vi "isValidCH.vi"(8 "error in":errorcluster, 10 "ValidCh":T2[](array[typedef]) items=["7"=7, "11"=11, "12"=12, "13"=13, "15"=15, "16"=16, "18"=18, "29"=29, "32"=32, "33"=33, "35"=35, "36"=36, "37"=37, "38"=38, "40"=40], 11 "CHStIn":T1) -> (0 "error out":errorcluster, 3 "VaildCH?":bool)   [LabVIEW 2014, in "ValveCTRL.lvlib"]
uses:
  ValveCTRL.lvlib
  TypeDef/CHs_List.ctl
  TypeDef/ChannelStatus.ctl
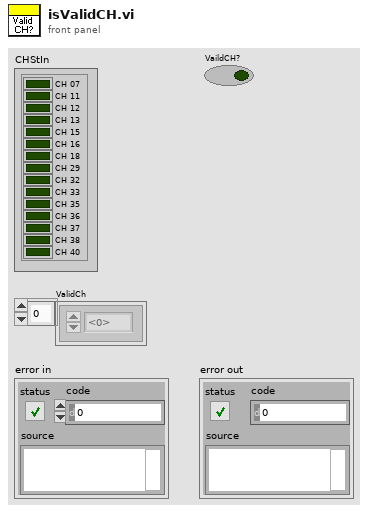
[diagram p1: front panel]
types:
  T1 = typedef "ValveCTRL.lvlib/ChannelStatus.ctl" = cluster{"CH 07":bool, "CH 11":bool, "CH 12":bool, "CH 13":bool, "CH 15":bool, "CH 16":bool, "CH 18":bool, "CH 29":bool, "CH 32":bool, "CH 33":bool, "CH 35":bool, "CH 36":bool, "CH 37":bool, "CH 38":bool, "CH 40":bool}
  T2 = typedef "ValveCTRL.lvlib/CHs_List.ctl" = u8
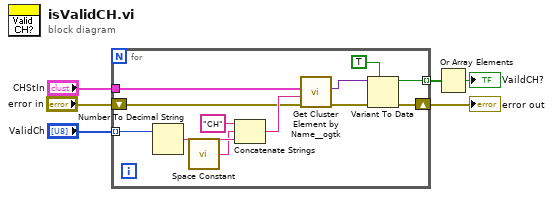
[diagram p0: block diagram]
diagram:
  n1 = for {
    tunnel: "ValidCh" -> [w17] mode=indexing
    tunnel: "CHStIn" -> [w18]
    shift-right: [w10] -> w2
    shift-left: "error in" -> [w12]
    tunnel: [w7] -> w4 mode=indexing
    n2 = Number To Decimal String(number=w17) -> (decimal integer string=w16:string)  [unwired: 1 in]
    n3 = call <vilib>:"Space Constant.vi"() -> ("String"=w15:string)
    n4 = Concatenate Strings("CH" ("string"), w15, w16) -> (w13:string)
    n5 = call <userlib>:"Get Cluster Element by Name__ogtk.vi"("error in (no error)"=w12, "Element Name"=w13, "Cluster"=w18) -> ("error out"=w11:errorcluster, "VElement"=w9:variant)  [unwired: 6 in, 1 out]
    n6 = Variant To Data(error in=w11, type=TRUE, Variant=w9) -> (data=w7:bool, error out=w10:errorcluster)
  }
  "error out" <- w2
  n7 = Or Array Elements(Boolean array=w4) -> (logical OR=→"VaildCH?":bool)
